vi "Insert temperature.vi"(1 "Temperature":dbl[unit]=273.15 format="%.1f", 2 "Sensor Data":T1 {"Sensor array"."scaled" format="%.2f"; "Sensor array"."voltage" format="%.4f"; "Time" format="%<%I:%M:%S%2u %p\n%m/%d/%Y>T"}) -> (0 "Sensor Data out":T1 {"Sensor array"."scaled" format="%.2f"; "Sensor array"."voltage" format="%.4f"; "Time" format="%<%I:%M:%S%2u %p\n%m/%d/%Y>T"})   [LabVIEW 2012]
uses:
  TCP DAQ/Sensor data.ctl
  DAQ configuration/sensor cluster.ctl
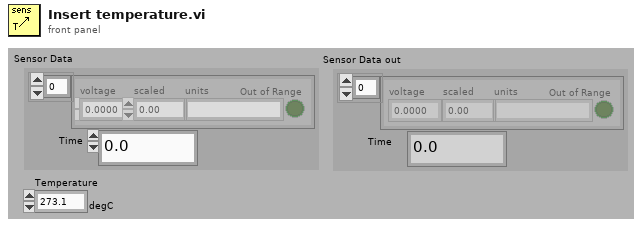
[diagram p1: front panel]
types:
  T1 = typedef "Sensor data.ctl" = cluster{" Sensor array":T2[], "Time":dbl}
  T2 = typedef "sensor cluster.ctl" = cluster{"voltage":sgl, "scaled":sgl, "units":string, "Out of Range":bool}
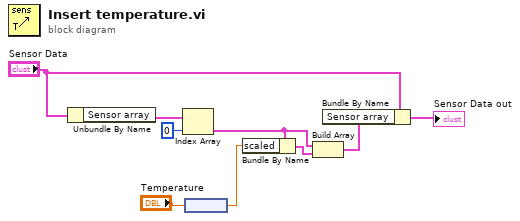
[diagram p0: block diagram]
diagram:
  n1 = Unbundle By Name("Sensor Data") -> ("Sensor array"=w7:T2[])
  n2 = Index Array(array=w7, index=0) -> (element=w3:T2)
  n3 = node("Temperature") -> (w4:dbl)
  n4 = Bundle By Name(cluster=w3, "scaled"=w4) -> (w2:T2)
  n5 = Build Array(w3, w2) -> (w1:T2[])
  n6 = Bundle By Name(cluster="Sensor Data", "Sensor array"=w1) -> (→"Sensor Data out":T1)
